vi "PPL_ActionVIOnRecompile.vi"(8 "error in":errorcluster, 9 "Timeout (ms)":u32, 10 "Runtime Configurable Section Path":string, 11 "Device Item Ref in":T1 format="%.0x") -> (0 "error out":errorcluster)   [LabVIEW 2020]
uses:
  <vilib>/NI VeriStand/Custom Device API/Custom Device Item Ref.ctl
  <vilib>/NI VeriStand/Custom Device API/Custom Device Channel Type.ctl
  <vilib>/NI VeriStand/Custom Device API/Data Access Type.ctl
  <vilib>/NI VeriStand/Execution/CustomDevice/NI VeriStand - Send Custom Device Message (Byte Array).vi
  <vilib>/NI VeriStand/Custom Device API/Custom Device API.lvlib
  <vilib>/NI VeriStand/Execution/CustomDevice/NI_VS Custom Device ExecutionAPI.lvlib
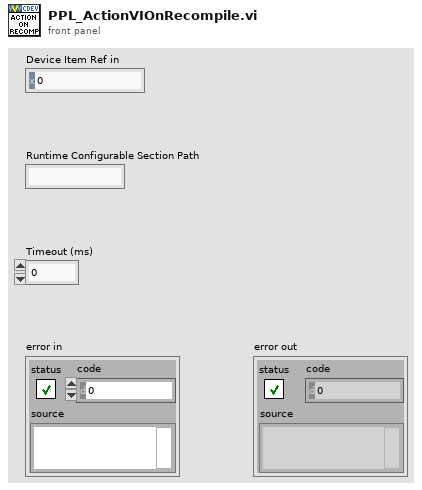
[diagram p1: front panel]
types:
  T1 = typedef "Custom Device API.lvlib/Custom Device Item Ref.ctl" = u64
  T2 = typedef "Custom Device API.lvlib/Custom Device Channel Type.ctl" = enum16{"Input", "Output"}
  T3 = typedef "Custom Device API.lvlib/Data Access Type.ctl" = enum16{"Read", "Write"}
  T4 = typedef "Custom Device API.lvlib/Custom Device Item Info.ctl" = cluster{"Name":string, "Is Channel":bool, "GUID":string, "Is Waveform":bool}
  T5 = typedef "NI_VS Custom Device ExecutionAPI.lvlib/Custom Device Ref.ctl" = refnum<k24>
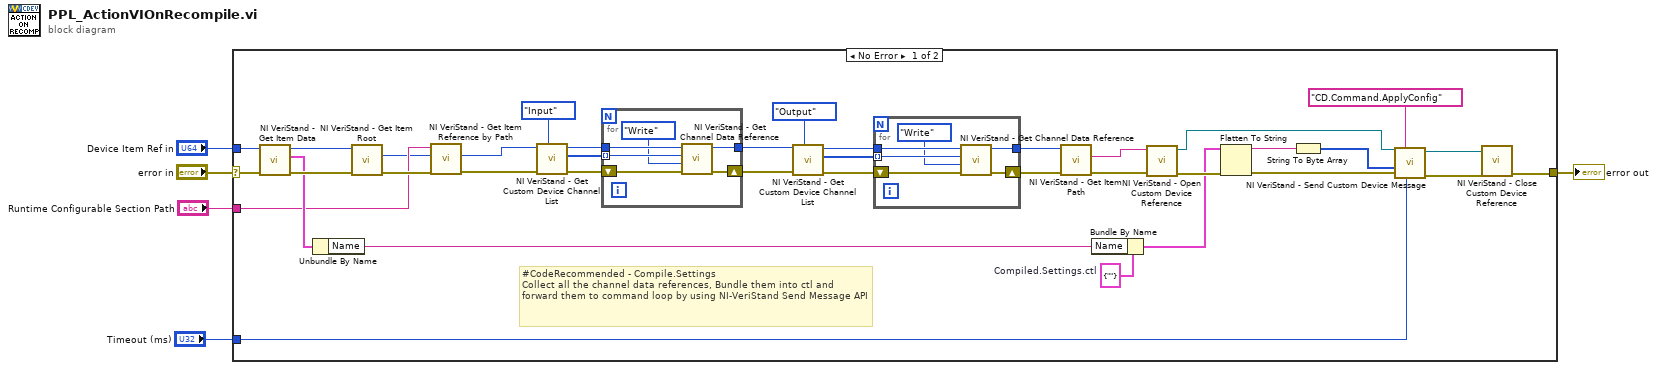
[diagram p0: block diagram]
diagram:
  n1 = case shown="No Error" "error in" {
    selector: "error in" -> [w42 w55]
    tunnel: [w31 w55] -> w4
    tunnel: "Device Item Ref in" -> [w29 _]
    tunnel: "Runtime Configurable Section Path" -> [w24 _]
    tunnel: "Timeout (ms)" -> [w7 _]
    frame No Error {
      w26 = cluster{"Name":string} {"Name"=""}  # Compiled.Settings.ctl
      # "#CodeRecommended - Compile.Settings\nCollect all the channel data references, Bundle them into ctl and forward them to command loop by using NI-VeriStand Send Message API"
      n2 = call <vilib>:"NI VeriStand - Get Item Data.vi"("error in (no error)"=w42, "Item Ref in"=w29) -> ("error out"=w41:errorcluster, "Item Info"=w28:T4, "Item Ref out"=w25:T1)  [unwired: 6 in, 1 out]
      n3 = Unbundle By Name(w28) -> ("Name"=w27:string)
      n4 = call <vilib>:"NI VeriStand - Get Item Root.vi"("error in (no error)"=w41, "Item Ref in"=w25) -> ("error out"=w40:errorcluster, "Root Ref out"=w23:T1)  [unwired: 6 in, 2 out]
      n5 = call <vilib>:"NI VeriStand - Get Item Reference by Path.vi"("error in (no error)"=w40, "Root Ref"=w23, "Item Path in"=w24) -> ("error out"=w39:errorcluster, "Item Ref"=w16:T1)  [unwired: 5 in, 2 out]
      n6 = call <vilib>:"NI VeriStand - Get Custom Device Channel List.vi"("Channel Type"=Custom_Device_Channel_Type."Input", "error in (no error)"=w39, "Device Ref in"=w16) -> ("error out"=w38:errorcluster, "Specified Channel Ref List"=w21:T1[], "Device Ref out"=w20:T1)  [unwired: 6 in]
      n7 = for {
        tunnel: w21 -> [w52] mode=indexing
        shift-right: [w53] -> w36
        shift-left: w38 -> [w54]
        tunnel: w20 -> [w51]
        tunnel: [w49] -> w15
        n8 = call <vilib>:"NI VeriStand - Get Channel Data Reference.vi"("error in (no error)"=w54, "Access"=Data_Access_Type."Write", "Channel Ref in"=w52, "Device Ref in"=w51) -> ("error out"=w53:errorcluster, "Device Ref out"=w49:T1)  [unwired: 5 in, 1 out]
      }
      n9 = call <vilib>:"NI VeriStand - Get Custom Device Channel List.vi"("Channel Type"=Custom_Device_Channel_Type."Output", "error in (no error)"=w36, "Device Ref in"=w15) -> ("error out"=w37:errorcluster, "Specified Channel Ref List"=w18:T1[], "Device Ref out"=w19:T1)  [unwired: 6 in]
      n10 = for {
        tunnel: w18 -> [w46] mode=indexing
        shift-right: [w47] -> w35
        shift-left: w37 -> [w48]
        tunnel: w19 -> [w45]
        tunnel: [w43] -> w14
        n11 = call <vilib>:"NI VeriStand - Get Channel Data Reference.vi"("error in (no error)"=w48, "Access"=Data_Access_Type."Write", "Channel Ref in"=w46, "Device Ref in"=w45) -> ("error out"=w47:errorcluster, "Device Ref out"=w43:T1)  [unwired: 5 in, 1 out]
      }
      n12 = call <vilib>:"NI VeriStand - Get Item Path.vi"("error in (no error)"=w35, "Item Ref in"=w14) -> ("error out"=w34:errorcluster, "Path"=w13:string)  [unwired: 6 in, 2 out]
      n13 = Bundle By Name(cluster=w26, "Name"=w27) -> (w12:cluster{"Name":string})
      n14 = call <vilib>:"NI VeriStand - Open Custom Device Reference.vi"("error in (no error)"=w34, "Custom Device Path"=w13) -> ("error out"=w33:errorcluster, "Custom Device"=w6:T5)  [unwired: 8 in]
      n15 = Flatten To String(anything=w12, error in (no error)=w33) -> (data string=w11:string, error out=w32:errorcluster)  [unwired: 2 in, 1 out]
      n16 = String To Byte Array(string=w11) -> (unsigned byte array=w10:u8[])
      n17 = call-poly <vilib>:"NI VeriStand - Send Custom Device Message.vi"("Timeout ms (5000)"=w7, "error in (no error)"=w32, "Data"=w10, "Command"="CD.Command.ApplyConfig", "Custom Device in"=w6) -> ("error out"=w30:errorcluster, "Custom Device out"=w8:T5)  [unwired: 4 in, 1 out]
      n18 = call <vilib>:"NI VeriStand - Close Custom Device Reference.vi"("error in (no error)"=w30, "Custom Device"=w8) -> ("error out"=w31:errorcluster)  [unwired: 9 in]
    }
    frame Error {
    }
  }
  "error out" <- w4
